vi "Create Item Name.vi"(6 "Parent":i32, 7 "Hide Full Name? (F)":bool, 10 "Type":variant, 11 "Item Graph In":T1[](array[typedef])) -> (2 "Name":string, 3 "Item Graph":T1[](array[typedef]))   [LabVIEW 2020, in "TypeGraph.lvlib"]
uses:
  TypeGraph.lvlib
  Type Reflection Item.ctl
  <vilib>/Utility/Data Type/NI_Data Type.lvlib
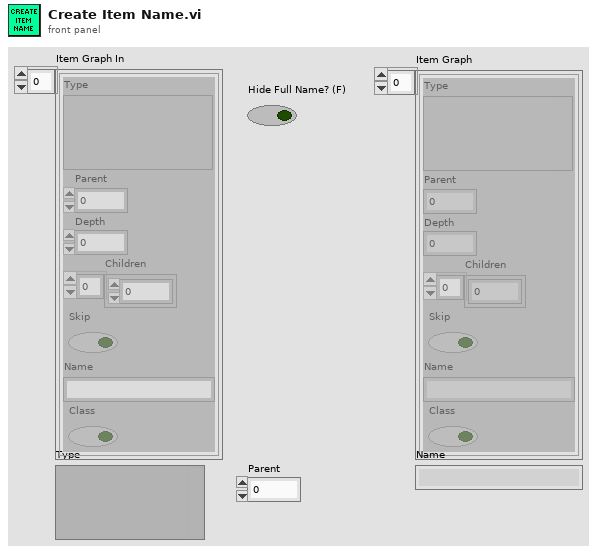
[diagram p1: front panel]
types:
  T1 = typedef "TypeGraph.lvlib/Type Reflection Item.ctl" = cluster{"Type":variant, "Parent":i32, "Depth":i32, "Children":i32[], "Skip":bool, "Name":string, "Class":bool}
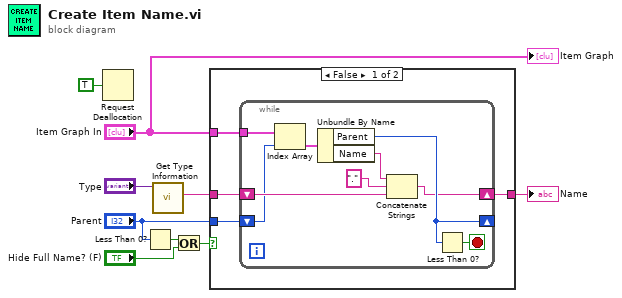
[diagram p0: block diagram]
diagram:
  n1 = Request Deallocation(TRUE ("flag")) -> ()
  n2 = Less Than 0?(x="Parent") -> (x < 0?=w6:bool)
  n3 = call <vilib>:"Get Type Information.vi"("variant"="Type") -> ("name"=w8:string)  [unwired: 6 in, 4 out]
  n4 = Or(x=w6, y="Hide Full Name? (F)") -> (x .or. y?=w4:bool)
  n5 = case shown="False" w4 {
    tunnel: w8 -> [w12 w23]
    tunnel: [w11 w23] -> w7
    tunnel: "Item Graph In" -> [w10 _]
    tunnel: "Parent" -> [w13 _]
    frame False {
      n6 = while {
        shift-right: [w19] -> _
        shift-left: w13 -> [w14]
        shift-right: [w15] -> w11
        shift-left: w12 -> [w18]
        tunnel: w10 -> [w21]
        stop <- w22 stop-if-true
        n7 = Index Array(array=w21, index=w14) -> (element=w20:T1)
        n8 = Unbundle By Name(w20) -> ("Parent"=w19:i32, "Name"=w17:string)
        n9 = Concatenate Strings(w17, "." ("string"), w18) -> (w15:string)
        n10 = Less Than 0?(x=w19) -> (x < 0?=w22:bool)
      }
    }
    frame True {
    }
  }
  "Name" <- w7
  "Item Graph" <- "Item Graph In"
